vi "Check Distance in Range.vi"(2 "Longitude Uncertainty":dbl=1e-05, 3 "Latitude Uncertainty":dbl=1e-05, 5 "Destination Longitude":dbl format="%#_9g", 6 "Destination Latitude":dbl format="%#_8g", 7 "Current Longitude":dbl format="%#_9g", 8 "Current Latitude":dbl format="%#_8g") -> (0 "Longitude Difference":dbl=2.6000000005410584e-05, 1 "Latitude Difference":dbl=2.200000000129876e-05, 4 "Distance in Range?":bool)   [LabVIEW 2011]
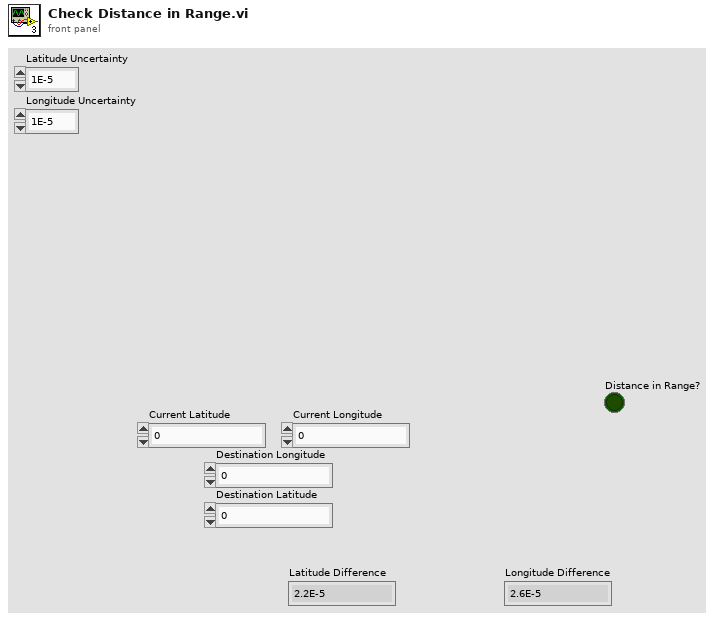
[diagram p1: front panel]
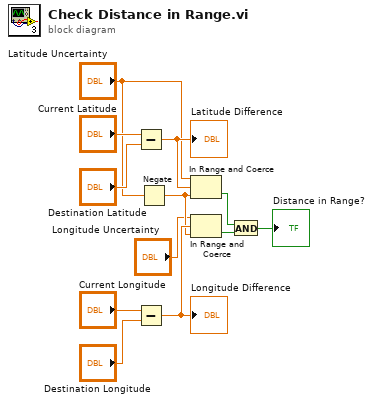
[diagram p0: block diagram]
diagram:
  n1 = Subtract(x="Current Latitude", y="Destination Latitude") -> (x-y=w10:dbl)
  "Latitude Difference" <- w10
  n2 = Subtract(x="Current Longitude", y="Destination Longitude") -> (x-y=w9:dbl)
  "Longitude Difference" <- w9
  n3 = Negate(x="Latitude Uncertainty") -> (-x=w3:dbl)
  n4 = In Range and Coerce(upper limit="Latitude Uncertainty", x=w10, lower limit=w3) -> (In Range?=w12:bool)  [unwired: 1 out]
  n5 = In Range and Coerce(upper limit="Longitude Uncertainty", x=w9, lower limit=w3) -> (In Range?=w11:bool)  [unwired: 1 out]
  n6 = And(x=w12, y=w11) -> (x .and. y?=→"Distance in Range?":bool)
